vi "SimpleAnyBuilder.vi"() -> ()   [LabVIEW 2019]
uses:
  labview source/Servers/Template Server/gRPC lvSupport/Server API/typeDefs/Message Element Type.ctl
  labview source/Servers/Template Server/gRPC lvSupport/Server API/typeDefs/Message Metadata.ctl
  labview source/Servers/Template Server/gRPC lvSupport/Server API/typeDefs/Message Element Metadata.ctl
  50cd6ca9-b915-40c5-a5da-5a0bdd109e0e.vi
  65d46b58-227a-49f8-b739-8ba8c807fa65.vi
  labview source/Servers/Template Server/gRPC lvSupport/Server API/Server/Get Server DLL Path.vi
  labview source/Servers/Template Server/gRPC lvSupport/gprc-lvsupport.lvlib
panel:
  out "Numeric":i32
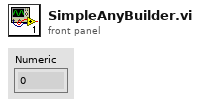
[diagram p1: front panel]
types:
  T1 = typedef "Template Server.lvlib/gprc-lvsupport.lvlib/Message Metadata.ctl" = cluster{"Version":i32, "Name":string, "Type Url":string, "Elements":T2[]}
  T2 = typedef "Template Server.lvlib/gprc-lvsupport.lvlib/Message Element Metadata.ctl" = cluster{"Embedded Message Name":string, "Protobuf Index":i32, "MessageElementType":T3, "Repeated":bool}
  T3 = typedef "Template Server.lvlib/gprc-lvsupport.lvlib/Message Element Type.ctl" = enum32{"Int32Value", "FloatValue", "DoubleValue", "BoolValue", "StringValue", "MessageValue", "Int64Value", "UInt32Value", "UInt64Value", "EnumValue"}
  T4 = typedef "Template Server.lvlib/gprc-lvsupport.lvlib/grpcId.ctl" = u64
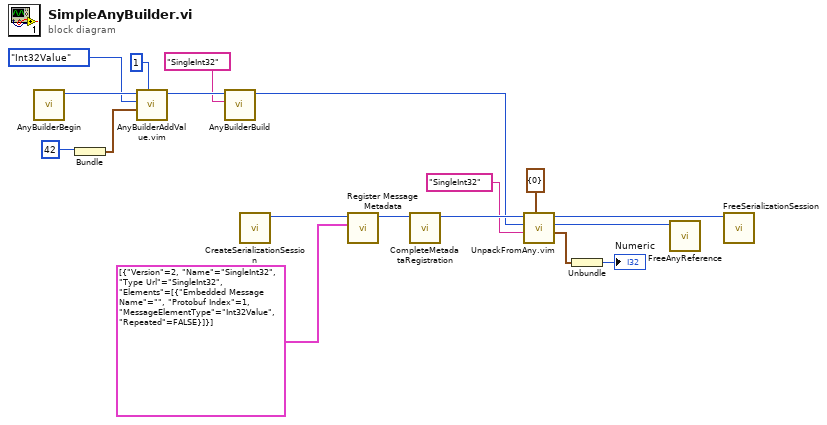
[diagram p0: block diagram]
diagram:
  n1 = call "AnyBuilderBegin.vi"() -> ("Builder Ref Out"=w18:T4)  [unwired: 9 in, 1 out]
  n2 = Bundle(42) -> (w15:cluster{i32})  [unwired: 1 in]
  n3 = call "AnyBuilderAddValue.vim"("protobufId"=1, "Value"=w15, "MessageElementType"=Message_Element_Type."Int32Value", "gRPCid in"=w18) -> ("gRPCid"=w13:u64)  [unwired: 6 in, 1 out]
  n4 = call "AnyBuilderBuild.vi"("Message Type"="SingleInt32", "Builder Ref"=w13) -> ("Any Reference Out"=w7:T4)  [unwired: 8 in, 1 out]
  n5 = call "CreateSerializationSession.vi"() -> ("Serialization Session ID"=w12:T4)  [unwired: 10 in, 1 out]
  n6 = call "Register Message Metadata.vi"("Messages"=T1[] [{"Version"=2, "Name"="SingleInt32", "Type Url"="SingleInt32", "Elements"=[{"Embedded Message Name"="", "Protobuf Index"=1, "MessageElementType"=enum."Int32Value", "Repeated"=FALSE}]}], "gRPCid"=w12) -> ("gRPCid"=w9:T4)  [unwired: 8 in, 1 out]
  n7 = call "CompleteMetadataRegistration.vi"("gRPC ID"=w9) -> ("gRPC ID Out"=w8:T4)  [unwired: 9 in, 1 out]
  n8 = call "UnpackFromAny.vim"("Data Type"=cluster{i32} {0}, "Message Type"="SingleInt32", "Any Reference in"=w7, "gRPCid in"=w8) -> ("Unpacked Value"=w4:cluster{i32}, "Any Reference Out"=w2:u64, "gRPCid"=w1:u64)  [unwired: 4 in, 1 out]
  n9 = Unbundle(w4) -> (→"Numeric":i32)
  n10 = call "FreeAnyReference.vi"("gRPCid in"=w2) -> ()  [unwired: 10 in, 1 out]
  n11 = call "FreeSerializationSession.vi"("Serialization Session ID"=w1) -> ()  [unwired: 10 in, 1 out]
